vi "ConvertDataDoubleToTaskStatus2.vi"(8 "error in (no error)":errorcluster, 9 "TaskStatus2":string(combo)="MaskValue", 10 "Double In":dbl[](array[numeric]), 11 "controller in":refnum<k24>) -> (0 "error out":errorcluster, 2 "TaskStatus2 Out":i32[](array[numeric]), 3 "controller out":refnum<k24>)   [LabVIEW 2010]
uses:
  c:/aerotech/controller/dev/A3200/pc/labview/2010/bin/Aerotech.A3200.dll
  bin/Aerotech.A3200.dll
  c:/aerotech/controller/dev/A3200/pc/labview/2010/bin/Aerotech.A3200.LabVIEW.dll
  bin/Aerotech.A3200.LabVIEW.dll
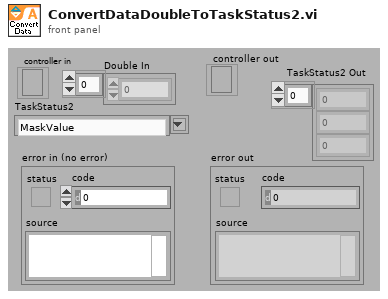
[diagram p1: front panel]
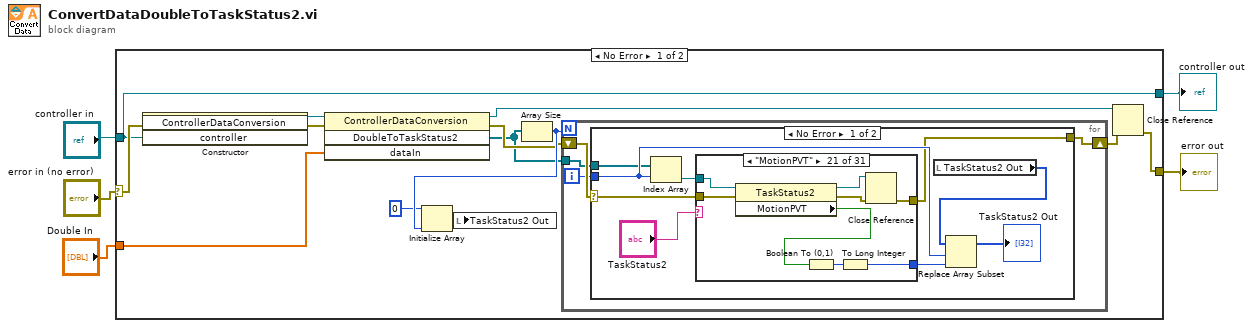
[diagram p0: block diagram]
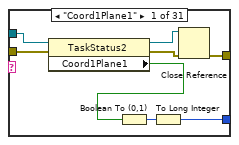
[diagram p2: hidden frame]
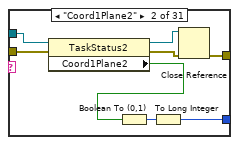
[diagram p3: hidden frame]
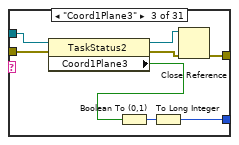
[diagram p4: hidden frame]
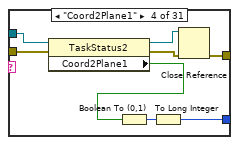
[diagram p5: hidden frame]
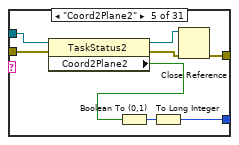
[diagram p6: hidden frame]
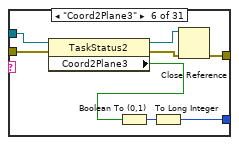
[diagram p7: hidden frame]
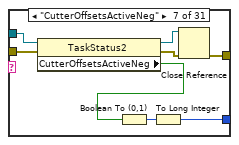
[diagram p8: hidden frame]
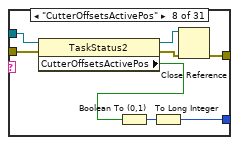
[diagram p9: hidden frame]
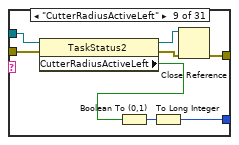
[diagram p10: hidden frame]
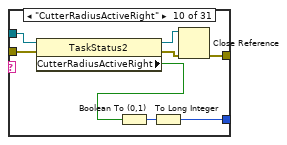
[diagram p11: hidden frame]
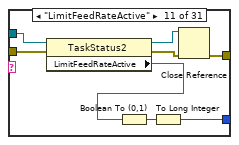
[diagram p12: hidden frame]
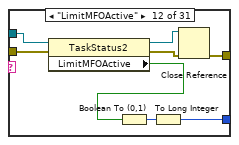
[diagram p13: hidden frame]
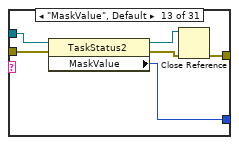
[diagram p14: hidden frame]
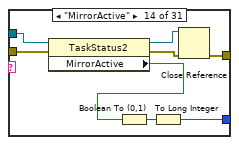
[diagram p15: hidden frame]
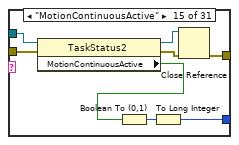
[diagram p16: hidden frame]
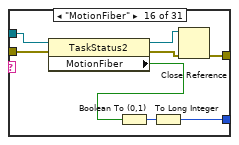
[diagram p17: hidden frame]
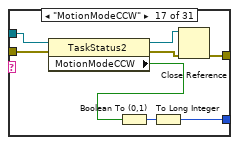
[diagram p18: hidden frame]
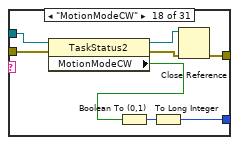
[diagram p19: hidden frame]
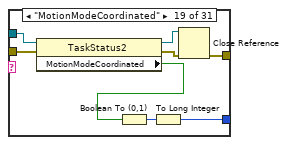
[diagram p20: hidden frame]
diagram:
  n1 = case shown="No Error" "error in (no error)" {
    selector: "error in (no error)" -> [w10 w280]
    tunnel: [w8 w280] -> w2
    tunnel: "controller in" -> [w7 w279]
    tunnel: "Double In" -> [w9 _]
    tunnel: [w7 w279] -> w1
    frame No Error {
      n2 = constructor class="ControllerDataConversion"(error in=w10, "controller"=w7) -> (reference out=w11:refnum<k24>, error out=w12:errorcluster)  [unwired: 2 in, 2 out]
      n3 = invoke class="ControllerDataConversion" method="DoubleToTaskStatus2"(reference=w11, error in=w12, "dataIn"=w9) -> (reference out=w13:refnum<k24>, error out=w15:errorcluster, "DoubleToTaskStatus2"=w14:refnum<k24>[])  [unwired: 1 in, 1 out]
      n4 = Array Size(array=w14) -> (size(s)=w18:i32)
      n5 = Initialize Array(0 ("element"), w18) -> (w6:i32[])
      n6 = local write "TaskStatus2 Out"(w6) -> ()
      n7 = for {
        N: w18 -> [_]
        tunnel: w14 -> [w20]
        shift-right: [w19] -> w16
        shift-left: w15 -> [w22]
        i -> [w21]
        n8 = case shown="No Error" w22 {
          selector: w22 -> [w26 w278]
          tunnel: [w23 w278] -> w19
          tunnel: w21 -> [w25 _]
          tunnel: w20 -> [w24 _]
          frame No Error {
            n9 = Index Array(array=w24, index=w25) -> (element=w31:refnum<k24>)
            n10 = case shown="\"MotionPVT\"" "TaskStatus2" {
              tunnel: w31 -> [w39 w47 w55 w63 w71 w79 w87 w95 w103 w111 w119 w127 w133 w141 w149 w157 w165 w173 w181 w189 w197 w205 w213 w221 w229 w237 w245 w253 w261 w269 w277]
              tunnel: w26 -> [w36 w44 w52 w60 w68 w76 w84 w92 w100 w108 w116 w124 w130 w138 w146 w154 w162 w170 w178 w186 w194 w202 w210 w218 w226 w234 w242 w250 w258 w266 w274]
              tunnel: [w34 w42 w50 w58 w66 w74 w82 w90 w98 w106 w114 w122 w128 w136 w144 w152 w160 w168 w176 w184 w192 w200 w208 w216 w224 w232 w240 w248 w256 w264 w272] -> w29
              tunnel: [w33 w41 w49 w57 w65 w73 w81 w89 w97 w105 w113 w121 w129 w135 w143 w151 w159 w167 w175 w183 w191 w199 w207 w215 w223 w231 w239 w247 w255 w263 w271] -> w23
              frame "Coord1Plane1" {
                n11 = property class="TaskStatus2"(reference=w39, error in=w36) -> (reference out=w38:refnum<k24>, error out=w37:errorcluster, "Coord1Plane1"=w32:bool)
                n12 = Boolean To (0,1)(Boolean=w32) -> (0, 1=w35:i16)
                n13 = To Long Integer(number=w35) -> (32bit integer=w34:i32)
                n14 = Close Reference(reference=w38, error in (no error)=w37) -> (error out=w33:errorcluster)
              }
              frame "Coord1Plane2" {
                n15 = property class="TaskStatus2"(reference=w47, error in=w44) -> (reference out=w46:refnum<k24>, error out=w45:errorcluster, "Coord1Plane2"=w40:bool)
                n16 = Boolean To (0,1)(Boolean=w40) -> (0, 1=w43:i16)
                n17 = To Long Integer(number=w43) -> (32bit integer=w42:i32)
                n18 = Close Reference(reference=w46, error in (no error)=w45) -> (error out=w41:errorcluster)
              }
              frame "Coord1Plane3" {
                n19 = property class="TaskStatus2"(reference=w55, error in=w52) -> (reference out=w54:refnum<k24>, error out=w53:errorcluster, "Coord1Plane3"=w48:bool)
                n20 = Boolean To (0,1)(Boolean=w48) -> (0, 1=w51:i16)
                n21 = To Long Integer(number=w51) -> (32bit integer=w50:i32)
                n22 = Close Reference(reference=w54, error in (no error)=w53) -> (error out=w49:errorcluster)
              }
              frame "Coord2Plane1" {
                n23 = property class="TaskStatus2"(reference=w63, error in=w60) -> (reference out=w62:refnum<k24>, error out=w61:errorcluster, "Coord2Plane1"=w56:bool)
                n24 = Boolean To (0,1)(Boolean=w56) -> (0, 1=w59:i16)
                n25 = To Long Integer(number=w59) -> (32bit integer=w58:i32)
                n26 = Close Reference(reference=w62, error in (no error)=w61) -> (error out=w57:errorcluster)
              }
              frame "Coord2Plane2" {
                n27 = property class="TaskStatus2"(reference=w71, error in=w68) -> (reference out=w70:refnum<k24>, error out=w69:errorcluster, "Coord2Plane2"=w64:bool)
                n28 = Boolean To (0,1)(Boolean=w64) -> (0, 1=w67:i16)
                n29 = To Long Integer(number=w67) -> (32bit integer=w66:i32)
                n30 = Close Reference(reference=w70, error in (no error)=w69) -> (error out=w65:errorcluster)
              }
              frame "Coord2Plane3" {
                n31 = property class="TaskStatus2"(reference=w79, error in=w76) -> (reference out=w78:refnum<k24>, error out=w77:errorcluster, "Coord2Plane3"=w72:bool)
                n32 = Boolean To (0,1)(Boolean=w72) -> (0, 1=w75:i16)
                n33 = To Long Integer(number=w75) -> (32bit integer=w74:i32)
                n34 = Close Reference(reference=w78, error in (no error)=w77) -> (error out=w73:errorcluster)
              }
              frame "CutterOffsetsActiveNeg" {
                n35 = property class="TaskStatus2"(reference=w87, error in=w84) -> (reference out=w86:refnum<k24>, error out=w85:errorcluster, "CutterOffsetsActiveNeg"=w80:bool)
                n36 = Boolean To (0,1)(Boolean=w80) -> (0, 1=w83:i16)
                n37 = To Long Integer(number=w83) -> (32bit integer=w82:i32)
                n38 = Close Reference(reference=w86, error in (no error)=w85) -> (error out=w81:errorcluster)
              }
              frame "CutterOffsetsActivePos" {
                n39 = property class="TaskStatus2"(reference=w95, error in=w92) -> (reference out=w94:refnum<k24>, error out=w93:errorcluster, "CutterOffsetsActivePos"=w88:bool)
                n40 = Boolean To (0,1)(Boolean=w88) -> (0, 1=w91:i16)
                n41 = To Long Integer(number=w91) -> (32bit integer=w90:i32)
                n42 = Close Reference(reference=w94, error in (no error)=w93) -> (error out=w89:errorcluster)
              }
              frame "CutterRadiusActiveLeft" {
                n43 = property class="TaskStatus2"(reference=w103, error in=w100) -> (reference out=w102:refnum<k24>, error out=w101:errorcluster, "CutterRadiusActiveLeft"=w96:bool)
                n44 = Boolean To (0,1)(Boolean=w96) -> (0, 1=w99:i16)
                n45 = To Long Integer(number=w99) -> (32bit integer=w98:i32)
                n46 = Close Reference(reference=w102, error in (no error)=w101) -> (error out=w97:errorcluster)
              }
              frame "CutterRadiusActiveRight" {
                n47 = property class="TaskStatus2"(reference=w111, error in=w108) -> (reference out=w110:refnum<k24>, error out=w109:errorcluster, "CutterRadiusActiveRight"=w104:bool)
                n48 = Boolean To (0,1)(Boolean=w104) -> (0, 1=w107:i16)
                n49 = To Long Integer(number=w107) -> (32bit integer=w106:i32)
                n50 = Close Reference(reference=w110, error in (no error)=w109) -> (error out=w105:errorcluster)
              }
              frame "LimitFeedRateActive" {
                n51 = property class="TaskStatus2"(reference=w119, error in=w116) -> (reference out=w118:refnum<k24>, error out=w117:errorcluster, "LimitFeedRateActive"=w112:bool)
                n52 = Boolean To (0,1)(Boolean=w112) -> (0, 1=w115:i16)
                n53 = To Long Integer(number=w115) -> (32bit integer=w114:i32)
                n54 = Close Reference(reference=w118, error in (no error)=w117) -> (error out=w113:errorcluster)
              }
              frame "LimitMFOActive" {
                n55 = property class="TaskStatus2"(reference=w127, error in=w124) -> (reference out=w126:refnum<k24>, error out=w125:errorcluster, "LimitMFOActive"=w120:bool)
                n56 = Boolean To (0,1)(Boolean=w120) -> (0, 1=w123:i16)
                n57 = To Long Integer(number=w123) -> (32bit integer=w122:i32)
                n58 = Close Reference(reference=w126, error in (no error)=w125) -> (error out=w121:errorcluster)
              }
              frame "MaskValue", Default {
                n59 = property class="TaskStatus2"(reference=w133, error in=w130) -> (reference out=w132:refnum<k24>, error out=w131:errorcluster, "MaskValue"=w128:i32)
                n60 = Close Reference(reference=w132, error in (no error)=w131) -> (error out=w129:errorcluster)
              }
              frame "MirrorActive" {
                n61 = property class="TaskStatus2"(reference=w141, error in=w138) -> (reference out=w140:refnum<k24>, error out=w139:errorcluster, "MirrorActive"=w134:bool)
                n62 = Boolean To (0,1)(Boolean=w134) -> (0, 1=w137:i16)
                n63 = To Long Integer(number=w137) -> (32bit integer=w136:i32)
                n64 = Close Reference(reference=w140, error in (no error)=w139) -> (error out=w135:errorcluster)
              }
              frame "MotionContinuousActive" {
                n65 = property class="TaskStatus2"(reference=w149, error in=w146) -> (reference out=w148:refnum<k24>, error out=w147:errorcluster, "MotionContinuousActive"=w142:bool)
                n66 = Boolean To (0,1)(Boolean=w142) -> (0, 1=w145:i16)
                n67 = To Long Integer(number=w145) -> (32bit integer=w144:i32)
                n68 = Close Reference(reference=w148, error in (no error)=w147) -> (error out=w143:errorcluster)
              }
              frame "MotionFiber" {
                n69 = property class="TaskStatus2"(reference=w157, error in=w154) -> (reference out=w156:refnum<k24>, error out=w155:errorcluster, "MotionFiber"=w150:bool)
                n70 = Boolean To (0,1)(Boolean=w150) -> (0, 1=w153:i16)
                n71 = To Long Integer(number=w153) -> (32bit integer=w152:i32)
                n72 = Close Reference(reference=w156, error in (no error)=w155) -> (error out=w151:errorcluster)
              }
              frame "MotionModeCCW" {
                n73 = property class="TaskStatus2"(reference=w165, error in=w162) -> (reference out=w164:refnum<k24>, error out=w163:errorcluster, "MotionModeCCW"=w158:bool)
                n74 = Boolean To (0,1)(Boolean=w158) -> (0, 1=w161:i16)
                n75 = To Long Integer(number=w161) -> (32bit integer=w160:i32)
                n76 = Close Reference(reference=w164, error in (no error)=w163) -> (error out=w159:errorcluster)
              }
              frame "MotionModeCW" {
                n77 = property class="TaskStatus2"(reference=w173, error in=w170) -> (reference out=w172:refnum<k24>, error out=w171:errorcluster, "MotionModeCW"=w166:bool)
                n78 = Boolean To (0,1)(Boolean=w166) -> (0, 1=w169:i16)
                n79 = To Long Integer(number=w169) -> (32bit integer=w168:i32)
                n80 = Close Reference(reference=w172, error in (no error)=w171) -> (error out=w167:errorcluster)
              }
              frame "MotionModeCoordinated" {
                n81 = property class="TaskStatus2"(reference=w181, error in=w178) -> (reference out=w180:refnum<k24>, error out=w179:errorcluster, "MotionModeCoordinated"=w174:bool)
                n82 = Boolean To (0,1)(Boolean=w174) -> (0, 1=w177:i16)
                n83 = To Long Integer(number=w177) -> (32bit integer=w176:i32)
                n84 = Close Reference(reference=w180, error in (no error)=w179) -> (error out=w175:errorcluster)
              }
              frame "MotionModeRapid" {
                n85 = property class="TaskStatus2"(reference=w189, error in=w186) -> (reference out=w188:refnum<k24>, error out=w187:errorcluster, "MotionModeRapid"=w182:bool)
                n86 = Boolean To (0,1)(Boolean=w182) -> (0, 1=w185:i16)
                n87 = To Long Integer(number=w185) -> (32bit integer=w184:i32)
                n88 = Close Reference(reference=w188, error in (no error)=w187) -> (error out=w183:errorcluster)
              }
              frame "MotionPVT" {
                n89 = property class="TaskStatus2"(reference=w197, error in=w194) -> (reference out=w196:refnum<k24>, error out=w195:errorcluster, "MotionPVT"=w190:bool)
                n90 = Boolean To (0,1)(Boolean=w190) -> (0, 1=w193:i16)
                n91 = To Long Integer(number=w193) -> (32bit integer=w192:i32)
                n92 = Close Reference(reference=w196, error in (no error)=w195) -> (error out=w191:errorcluster)
              }
              frame "None" {
                n93 = property class="TaskStatus2"(reference=w205, error in=w202) -> (reference out=w204:refnum<k24>, error out=w203:errorcluster, "None"=w198:bool)
                n94 = Boolean To (0,1)(Boolean=w198) -> (0, 1=w201:i16)
                n95 = To Long Integer(number=w201) -> (32bit integer=w200:i32)
                n96 = Close Reference(reference=w204, error in (no error)=w203) -> (error out=w199:errorcluster)
              }
              frame "NormalcyActiveLeft" {
                n97 = property class="TaskStatus2"(reference=w213, error in=w210) -> (reference out=w212:refnum<k24>, error out=w211:errorcluster, "NormalcyActiveLeft"=w206:bool)
                n98 = Boolean To (0,1)(Boolean=w206) -> (0, 1=w209:i16)
                n99 = To Long Integer(number=w209) -> (32bit integer=w208:i32)
                n100 = Close Reference(reference=w212, error in (no error)=w211) -> (error out=w207:errorcluster)
              }
              frame "NormalcyActiveRight" {
                n101 = property class="TaskStatus2"(reference=w221, error in=w218) -> (reference out=w220:refnum<k24>, error out=w219:errorcluster, "NormalcyActiveRight"=w214:bool)
                n102 = Boolean To (0,1)(Boolean=w214) -> (0, 1=w217:i16)
                n103 = To Long Integer(number=w217) -> (32bit integer=w216:i32)
                n104 = Close Reference(reference=w220, error in (no error)=w219) -> (error out=w215:errorcluster)
              }
              frame "NormalcyAlignment" {
                n105 = property class="TaskStatus2"(reference=w229, error in=w226) -> (reference out=w228:refnum<k24>, error out=w227:errorcluster, "NormalcyAlignment"=w222:bool)
                n106 = Boolean To (0,1)(Boolean=w222) -> (0, 1=w225:i16)
                n107 = To Long Integer(number=w225) -> (32bit integer=w224:i32)
                n108 = Close Reference(reference=w228, error in (no error)=w227) -> (error out=w223:errorcluster)
              }
              frame "OffsetFixtureActive" {
                n109 = property class="TaskStatus2"(reference=w237, error in=w234) -> (reference out=w236:refnum<k24>, error out=w235:errorcluster, "OffsetFixtureActive"=w230:bool)
                n110 = Boolean To (0,1)(Boolean=w230) -> (0, 1=w233:i16)
                n111 = To Long Integer(number=w233) -> (32bit integer=w232:i32)
                n112 = Close Reference(reference=w236, error in (no error)=w235) -> (error out=w231:errorcluster)
              }
              frame "ProfileActive" {
                n113 = property class="TaskStatus2"(reference=w245, error in=w242) -> (reference out=w244:refnum<k24>, error out=w243:errorcluster, "ProfileActive"=w238:bool)
                n114 = Boolean To (0,1)(Boolean=w238) -> (0, 1=w241:i16)
                n115 = To Long Integer(number=w241) -> (32bit integer=w240:i32)
                n116 = Close Reference(reference=w244, error in (no error)=w243) -> (error out=w239:errorcluster)
              }
              frame "RThetaCylindricalActive" {
                n117 = property class="TaskStatus2"(reference=w253, error in=w250) -> (reference out=w252:refnum<k24>, error out=w251:errorcluster, "RThetaCylindricalActive"=w246:bool)
                n118 = Boolean To (0,1)(Boolean=w246) -> (0, 1=w249:i16)
                n119 = To Long Integer(number=w249) -> (32bit integer=w248:i32)
                n120 = Close Reference(reference=w252, error in (no error)=w251) -> (error out=w247:errorcluster)
              }
              frame "RThetaPolarActive" {
                n121 = property class="TaskStatus2"(reference=w261, error in=w258) -> (reference out=w260:refnum<k24>, error out=w259:errorcluster, "RThetaPolarActive"=w254:bool)
                n122 = Boolean To (0,1)(Boolean=w254) -> (0, 1=w257:i16)
                n123 = To Long Integer(number=w257) -> (32bit integer=w256:i32)
                n124 = Close Reference(reference=w260, error in (no error)=w259) -> (error out=w255:errorcluster)
              }
              frame "RotationActive" {
                n125 = property class="TaskStatus2"(reference=w269, error in=w266) -> (reference out=w268:refnum<k24>, error out=w267:errorcluster, "RotationActive"=w262:bool)
                n126 = Boolean To (0,1)(Boolean=w262) -> (0, 1=w265:i16)
                n127 = To Long Integer(number=w265) -> (32bit integer=w264:i32)
                n128 = Close Reference(reference=w268, error in (no error)=w267) -> (error out=w263:errorcluster)
              }
              frame "ScalingActive" {
                n129 = property class="TaskStatus2"(reference=w277, error in=w274) -> (reference out=w276:refnum<k24>, error out=w275:errorcluster, "ScalingActive"=w270:bool)
                n130 = Boolean To (0,1)(Boolean=w270) -> (0, 1=w273:i16)
                n131 = To Long Integer(number=w273) -> (32bit integer=w272:i32)
                n132 = Close Reference(reference=w276, error in (no error)=w275) -> (error out=w271:errorcluster)
              }
            }
            n133 = local read "TaskStatus2 Out"() -> (w27:i32[])
            n134 = Replace Array Subset(array=w27, new element=w29, index=w25) -> (→"TaskStatus2 Out":i32[])
          }
          frame Error {
          }
        }
      }
      n135 = Close Reference(reference=w13, error in (no error)=w16) -> (error out=w8:errorcluster)
    }
    frame Error {
    }
  }
  "error out" <- w2
  "controller out" <- w1
